vi "Write DAQ Data.vi"(8 "error in (no error)":errorcluster, 9 "Voltage with Time":dbl[][](array[numeric]), 10 "File Infor":T1, 11 "TDMS File in":refnum<class "TDMS File.lvclass">) -> (0 "error out":errorcluster, 3 "TDMS File out":refnum<class "TDMS File.lvclass">)   [LabVIEW 2021, in "TDMS File.lvclass"]
doc: "This vi helps to write Voltage with Time 2 dimensional array into TDMS file."
uses:
  TDMS File.lvclass
  Control/File Information Cluster.ctl
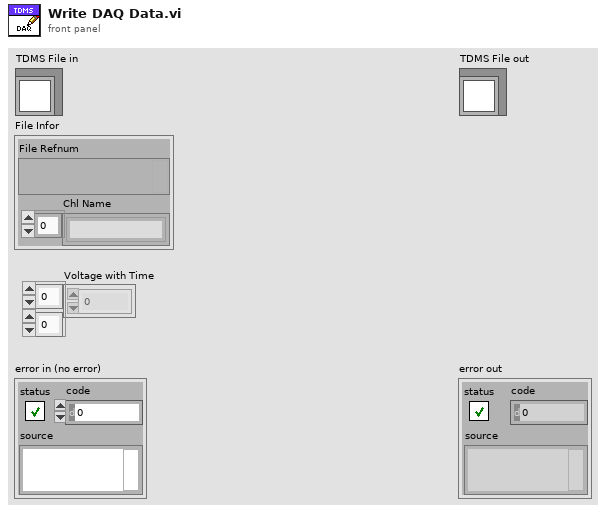
[diagram p1: front panel]
types:
  T1 = typedef "File Information Cluster.ctl" = cluster{"File Refnum":variant, "Chl Name":string[]}
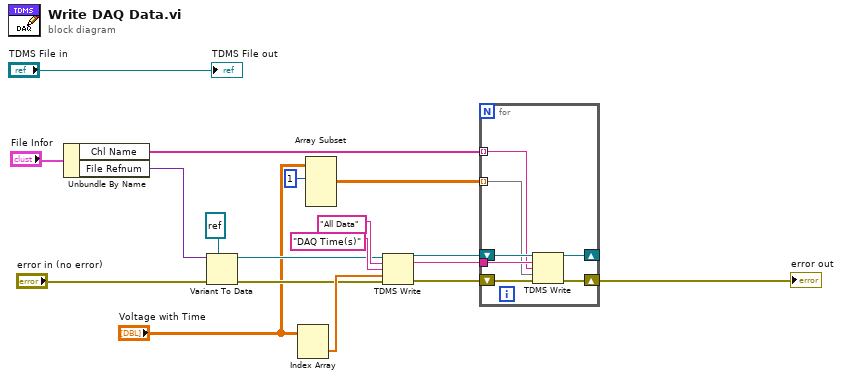
[diagram p0: block diagram]
diagram:
  n1 = Unbundle By Name("File Infor") -> ("Chl Name"=w3:string[], "File Refnum"=w6:variant)
  n2 = Variant To Data(error in="error in (no error)", type=refnum<k34> refnum ("tdms Refnum"), Variant=w6) -> (data=w8:refnum<k34>, error out=w7:errorcluster)
  n3 = Index Array(array="Voltage with Time") -> (element=w16:dbl[])  [unwired: 2 in]
  n4 = Array Subset(array="Voltage with Time", index (row)=1 ("index")) -> (w12:dbl[][])  [unwired: 3 in]
  n5 = TDMS Write(0:w8, 5:"All Data" ("group name in (Untitled)"), 7:"DAQ Time(s)", 9:w16, 11:w7) -> (4:w13:refnum<k34>, 6:w14:string, 15:w11:errorcluster)  [unwired: 1 in, 1 out]
  n6 = for {
    tunnel: w14 -> [w25]
    tunnel: w12 -> [w23] mode=indexing
    shift-right: [w21] -> _
    shift-left: w13 -> [w24]
    shift-right: [w20] -> w10
    shift-left: w11 -> [w22]
    tunnel: w3 -> [w19] mode=indexing
    n7 = TDMS Write(0:w24, 5:w25, 7:w19, 9:w23, 11:w22) -> (4:w21:refnum<k34>, 15:w20:errorcluster)  [unwired: 1 in, 2 out]
  }
  "error out" <- w10
  "TDMS File out" <- "TDMS File in"
